vi "Do.vi"(8 "error in (no error)":errorcluster, 10 "Actor in":refnum<class "Actor.lvclass">, 11 "Register Instrument Msg":refnum<class "Register Instrument Msg.lvclass">) -> (0 "error out":errorcluster, 2 "Actor out":refnum<class "Actor.lvclass">)   [LabVIEW 2020, in "Instrument Handler.lvlib" / "Register Instrument Msg.lvclass"]
doc: "This implementation calls the 'Register Instrument' method on the Instrument Handler."
uses:
  Register Instrument Msg.lvclass
  PPL/HDH.Actor Framework.Core.Actor.lvlibp/1abvi3w/vi.lib/ActorFramework/Actor/Actor.lvclass
  Instrument Handler/Instrument Handler.lvclass
  C:/Current projects/WS/PPL/HDH.Actor Framework.Core.Actor.lvlibp/1abvi3w/vi.lib/ActorFramework/Actor/Actor.lvclass
  Register Instrument Msg.lvclass/Register Instrument Msg.ctl
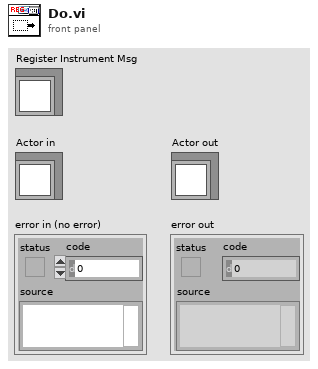
[diagram p1: front panel]
types:
  T1 = typedef "HDH.Actor Framework.Core.Instrument Driver.lvlibp/Instrument Driver.lvclass/Ctl_ConnectionType.ctl" = enum16{"BuiltIn/System", "PXI/PCI", "USB", "GPIB", "VXI", "Serial", "TCP/IP", "cRIO", "SCXI", "cDAQ", "SwitchBlock", "SCC", "FireWire", "Accessory", "CAN", "SwitchBlock Device"}
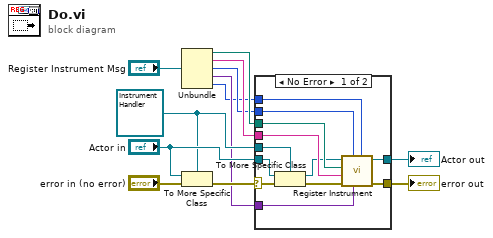
[diagram p0: block diagram]
diagram:
  w6 = refnum<class "Instrument Handler.lvclass"> refnum ("Actor in")
  n1 = Unbundle("Register Instrument Msg") -> (w5:path, w4:string, w3:T1, w2:variant, w1:u32)
  n2 = To More Specific Class(target class=w6, reference="Actor in", error in="error in (no error)") -> (error out=w10:errorcluster)  [unwired: 1 out]
  n3 = case shown="No Error" w10 {
    selector: w10 -> [w15 w26]
    tunnel: [w24 w26] -> w9
    tunnel: [w23 w25] -> w8
    tunnel: "Actor in" -> [w22 w25]
    tunnel: w6 -> [w21 _]
    tunnel: w5 -> [w19 _]
    tunnel: w4 -> [w18 _]
    tunnel: w3 -> [w17 _]
    tunnel: w2 -> [w20 _]
    tunnel: w1 -> [w13 _]
    frame No Error {
      n4 = To More Specific Class(target class=w21, reference=w22, error in=w15) -> (specific class reference=w16:refnum<class "Instrument Handler.lvclass">, error out=w14:errorcluster)
      n5 = call "Register Instrument.vi"("Instrument ID"=w13, "Pre Initialization Data"=w20, "Connection Type"=w17, "error in (no error)"=w14, "Alias"=w18, "Driver Path"=w19, "Instrument Handler in"=w16) -> ("error out"=w24:errorcluster, "Instrument Handler out"=w23:refnum<class "Instrument Handler.lvclass">)  [unwired: 3 in]
    }
    frame Error {
    }
  }
  "error out" <- w9
  "Actor out" <- w8
